vi "process time convertion.vi"(1 "process_time":u32) -> (0 "out":string)   [LabVIEW 2012]
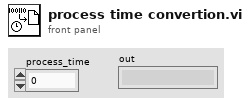
[diagram p1: front panel]
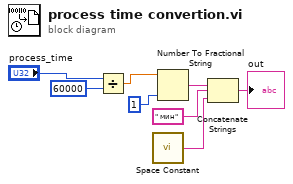
[diagram p0: block diagram]
diagram:
  n1 = Divide(x="process_time", y=u32 60000) -> (x/y=w5:dbl)
  n2 = call <vilib>:"Space Constant.vi"() -> ("String"=w1:string)
  n3 = Number To Fractional String(number=w5, precision (6)=i16 1 ("width (-)")) -> (F-format string=w3:string)  [unwired: 2 in]
  n4 = Concatenate Strings(w3, " мин" ("string"), w1) -> (→"out":string)
